vi "UpdateNumberOfElement.vi"(8 "error in (no error)":errorcluster, 10 "Nb Element":u64, 11 "Progress in":refnum<class "Progress.lvclass">) -> (0 "error out":errorcluster, 3 "Progress out":refnum<class "Progress.lvclass">)   [LabVIEW 2021, in "Progress.lvlib" / "Progress.lvclass"]
uses:
  Progress.lvclass
  Progress.lvclass/Progress.ctl
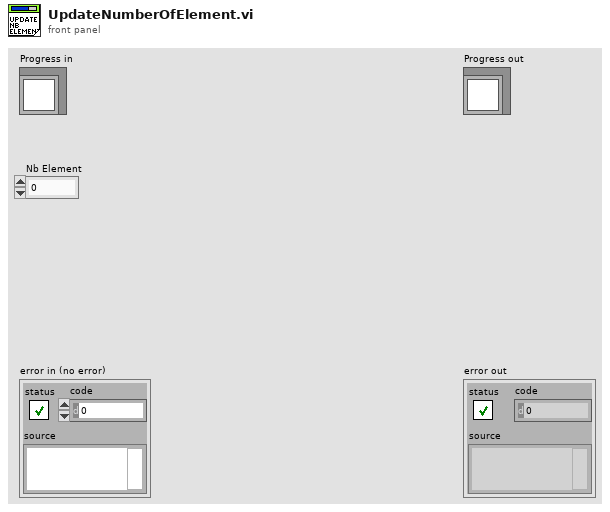
[diagram p1: front panel]
types:
  T1 = typedef "Progress.lvlib/Progress.lvclass/Data.ctl" = cluster{"SlideRefnum":refnum<vi>, "ProgressValue":u64, "NbElement":u64, "Caption":string, "UINotifier":refnum<notifier>, "StopUI":refnum<user-event>}
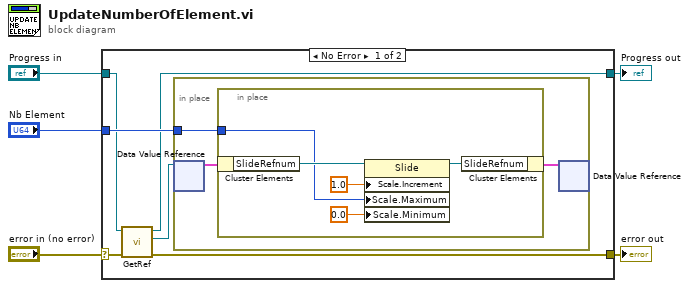
[diagram p0: block diagram]
diagram:
  n1 = case shown="No Error" "error in (no error)" {
    selector: "error in (no error)" -> [w11 w21]
    tunnel: [w9 w21] -> w4
    tunnel: [w7 w20] -> w2
    tunnel: "Progress in" -> [w8 w20]
    tunnel: "Nb Element" -> [w10 _]
    frame No Error {
      n2 = call "GetRef.vi"("error in (no error)"=w11, "Progress in"=w8) -> ("error out"=w9:errorcluster, "ref"=w6:refnum<data-value>, "Progress out"=w7:refnum<class "Progress.lvclass">)  [unwired: 7 in]
      n3 = in-place {
        in-place-border: w10 -> [w14]
        n4 = in-place-dvr #1(w6) -> (w13:T1)  [unwired: 1 out]
        n5 = in-place {
          in-place-border: w14 -> [w15]
          n6 = in-place-cluster #2(w13) -> ("SlideRefnum"=w19:refnum<vi>)
          n7 = property class="Slide"(reference=w19, "Scale.Increment"=1.0 ("Scale.Range:Increment"), "Scale.Maximum"=w15, "Scale.Minimum"=0.0 ("ProgressValue")) -> (reference out=w18:refnum<vi>)  [unwired: 1 in, 1 out]
          n8 = in-place-cluster #2("SlideRefnum"=w18) -> (w12:T1)
        }
        n9 = in-place-dvr #1(w12) -> ()  [unwired: 2 out]
      }
    }
    frame Error {
    }
  }
  "error out" <- w4
  "Progress out" <- w2
